vi "Demo.vi"(9 "beta 2":dbl(slide)=137.76536312849163 scale=-180.0..180.0, 10 "beta 1":dbl(slide)=43.24022346368716 scale=-180.0..180.0) -> ()   [LabVIEW 2020]
uses:
  arm/onshape/Onshape/WriteOnshapeAngle.vi
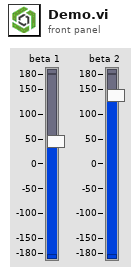
[diagram p1: front panel]
types:
  T1 = cluster{"did":string, "wid":string, "eid":string}
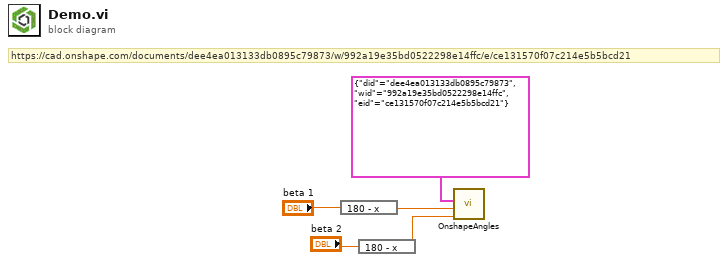
[diagram p0: block diagram]
diagram:
  # "https://cad.onshape.com/documents/dee4ea013133db0895c79873/w/992a19e35bd0522298e14ffc/e/ce131570f07c214e5b5bcd21"
  n1 = expression code="180 - x"("beta 1") -> (w2:dbl)
  n2 = expression code="180 - x"("beta 2") -> (w1:dbl)
  n3 = call-poly "OnshapeAngles.vi"("Angle2In"=w1, "Angle1In"=w2, "IDs"=T1 {"did"="dee4ea013133db0895c79873", "wid"="992a19e35bd0522298e14ffc", "eid"="ce131570f07c214e5b5bcd21"}) -> ()  [unwired: 8 in, 1 out]
